vi "Write Digital Bits.vi"(8 "error in":errorcluster, 9 "Bits:":bool[](array[boolean]), 10 "Memory Start:":u16, 11 "MiniIO in":refnum<class "MiniIO.lvclass">) -> (0 "error out":errorcluster, 3 "MiniIO out":refnum<class "MiniIO.lvclass">)   [LabVIEW 2018, in "MiniIO.lvlib" / "MiniIO.lvclass"]
doc: "Write to Digital Bits. This is used to write digital outputs or Blink mode bits to the Mini IO.\n\nMemory start locations are: \n\n200 for Digital Output\n300 for Blinking Output"
uses:
  MiniIO.lvclass
  MiniIO.lvclass/MiniIO.ctl
  <vilib>/NI/Modbus Library/API/Master/Modbus Master.lvclass
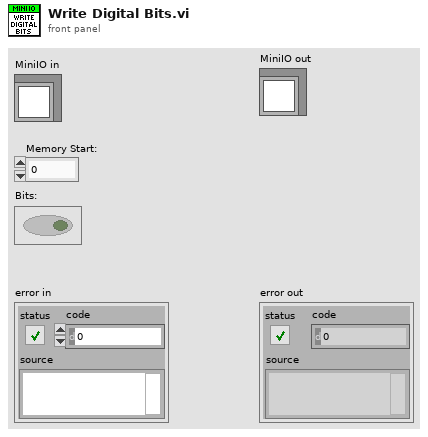
[diagram p1: front panel]
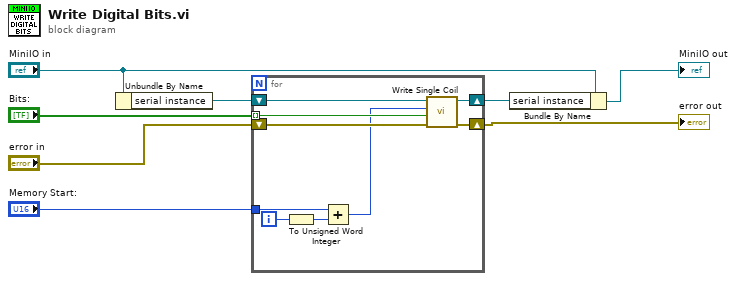
[diagram p0: block diagram]
diagram:
  n1 = Unbundle By Name("MiniIO in") -> ("serial instance"=w5:refnum<class "Modbus Master.lvclass">)
  n2 = for {
    shift-right: [w16] -> w1
    shift-left: w5 -> [w17]
    tunnel: "Memory Start:" -> [w15]
    shift-right: [w14] -> w3
    shift-left: "error in" -> [w13]
    tunnel: "Bits:" -> [w12] mode=indexing
    i -> [w10]
    n3 = To Unsigned Word Integer(number=w10) -> (unsigned 16bit integer=w9:u16)
    n4 = Add(x=w15, y=w9) -> (x+y=w11:u16)
    n5 = call-dynamic "Write Single Coil.vi"("error in"=w13, "coil to write"=w12, "address"=w11, "Modbus master in"=w17) -> ("error out"=w14:errorcluster, "Modbus master out"=w16:refnum<class "Modbus Master.lvclass">)  [unwired: 6 in]
  }
  "error out" <- w3
  n6 = Bundle By Name(cluster="MiniIO in", "serial instance"=w1) -> (→"MiniIO out":refnum<class "MiniIO.lvclass">)
